vi "Get Elements Inside Reference By Type.vi"(8 "error in (no error)":errorcluster, 10 "filter element class name":string, 11 "element ref.":refnum<vi>) -> (0 "error out":errorcluster, 2 "elemnts count":i32, 3 "elements ref.":refnum<vi>[](array[refnum]))   [LabVIEW 2018]
doc: "Returns referencies and UIDs of elements specified by ClassName which are children of wired element."
uses:
  <vilib>/Utility/traverseref.llb/TRef TravTarget.ctl
  <vilib>/Utility/traverseref.llb/VI Scripting - Traverse.lvlib
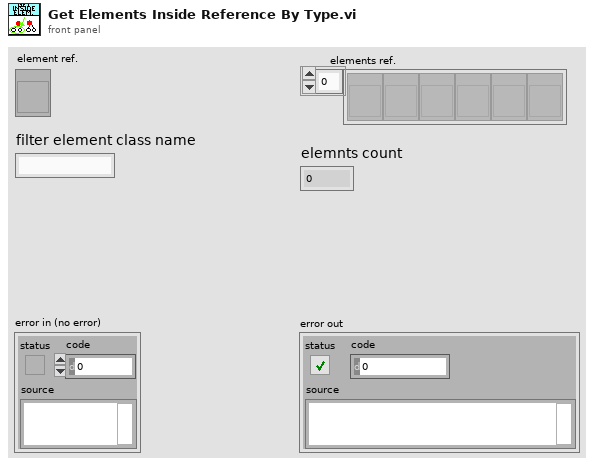
[diagram p1: front panel]
types:
  T1 = typedef "TRef TravTarget.ctl" = enum16{"FP", "BD", "Other"}
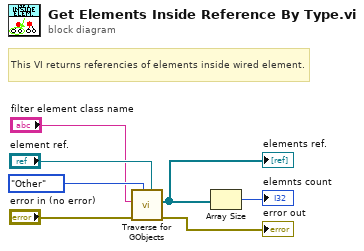
[diagram p0: block diagram]
diagram:
  # "This VI returns referencies of elements inside wired element."
  n1 = call <vilib>:"Traverse for GObjects.vi"("Other Refnum"="element ref.", "Traverse Target"=TRef_TravTarget."Other", "error in (no error)"="error in (no error)", "Class Name"="filter element class name") -> ("error out"=→"error out":errorcluster, "References"=w1:refnum<vi>[])  [unwired: 4 in, 2 out]
  "elements ref." <- w1
  n2 = Array Size(array=w1) -> (size(s)=→"elemnts count":i32)
